vi "Get_PreviewCache.vi"(8 "error in (no error)":errorcluster, 11 "PreviewCache in":refnum<class "PreviewCache.lvclass">) -> (0 "error out":errorcluster, 2 "data":T1, 3 "PreviewCache out":refnum<class "PreviewCache.lvclass">)   [LabVIEW 2020, in "PreviewCache.lvclass"]
uses:
  <vilib>/AppBuilder/AB_Classes/PreviewCache/PreviewCache.lvclass
  <vilib>/AppBuilder/AB_Classes/PreviewCache/PreviewCache.ctl
  <vilib>/AppBuilder/AB_Classes/PreviewCache/build preview data.ctl
  <vilib>/AppBuilder/AB_Classes/PreviewCache/PreviewCache.lvclass/PreviewCache.ctl
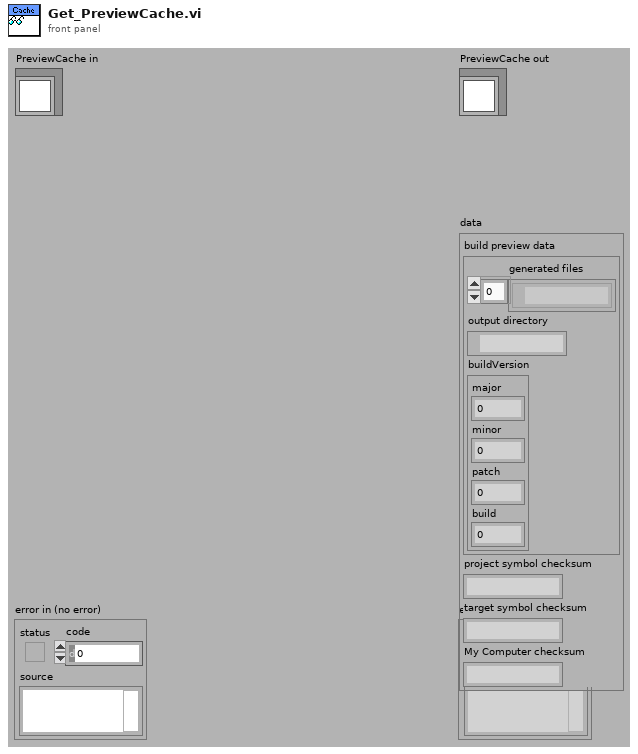
[diagram p1: front panel]
types:
  T1 = typedef "PreviewCache.ctl" = cluster{"build preview data":T2, "project symbol checksum":string, "target symbol checksum":string, "My Computer checksum":string}
  T2 = typedef "build preview data.ctl" = cluster{"generated files":path[], "output directory":path, "buildVersion":cluster{"major":u16, "minor":u16, "patch":u16, "build":u16}}
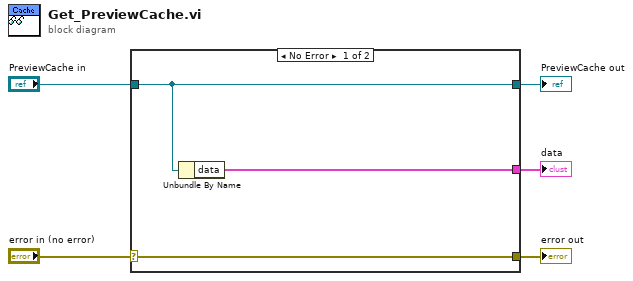
[diagram p0: block diagram]
diagram:
  n1 = case shown="No Error" "error in (no error)" {
    selector: "error in (no error)" -> [w8 w9]
    tunnel: [w8 w9] -> w4
    tunnel: [w7 w10] -> w2
    tunnel: "PreviewCache in" -> [w7 w10]
    tunnel: [w6 _] -> w1
    frame No Error {
      n2 = Unbundle By Name(w7) -> ("data"=w6:T1)
    }
    frame Error {
    }
  }
  "error out" <- w4
  "PreviewCache out" <- w2
  "data" <- w1
